vi "Write Plugin Type.vi"(8 "error in (no error)":errorcluster, 10 "Plugin Type":refnum<class>, 11 "Factory Plugin Framework in":refnum<class "Factory Plugin Framework.lvclass">=refnum) -> (0 "error out":errorcluster, 3 "Factory Plugin Framework out":refnum<class "Factory Plugin Framework.lvclass">)   [LabVIEW 2018, in "Factory Plugin Framework.lvlib" / "Factory Plugin Framework.lvclass"]
uses:
  Factory Plugin Framework.lvclass
  Factory Plugin Framework.lvclass/Factory Plugin Framework.ctl
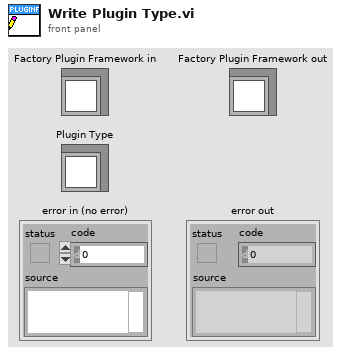
[diagram p1: front panel]
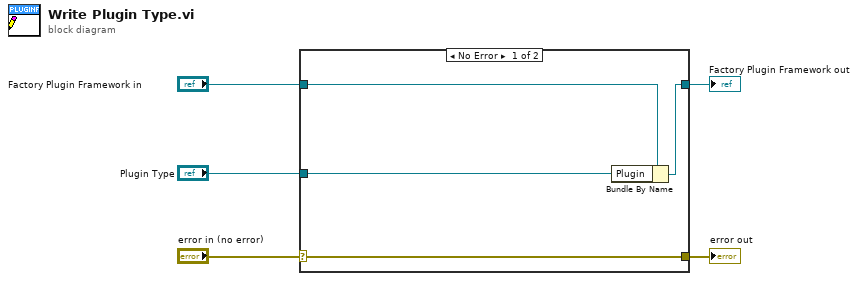
[diagram p0: block diagram]
diagram:
  n1 = case shown="No Error" "error in (no error)" {
    selector: "error in (no error)" -> [w9 w10]
    tunnel: [w9 w10] -> w4
    tunnel: [w7 w11] -> w2
    tunnel: "Factory Plugin Framework in" -> [w8 w11]
    tunnel: "Plugin Type" -> [w6 _]
    frame No Error {
      n2 = Bundle By Name(cluster=w8, "Plugin"=w6) -> (w7:refnum<class "Factory Plugin Framework.lvclass">)
    }
    frame Error {
    }
  }
  "error out" <- w4
  "Factory Plugin Framework out" <- w2
